vi "בדיקת מפל מתח בין הדקי הממסר תחת עומס 7.vi"(8 "error":errorcluster, 11 "Path for Log":path) -> (0 "error IO":errorcluster, 1 "בטווח כן/לא":bool, 2 "מפל מתח בין דקי הממסר תחת עומס":dbl, 3 "תוצאה זמנית":dbl)   [LabVIEW 2014]
uses:
  M9700 Driver/85/vi.lib/M9700 Modbus.llb/CTL Register Address.ctl
  M9700 Driver/86/vi.lib/M9700 Modbus.llb/CTL CMD Register.ctl
  <vilib>/Instr/_visa.llb/VISA Configure Serial Port (Instr).vi
  <vilib>/DAQmx/create/channels.llb/DAQmx Create Channel (DO-Digital Output).vi
  <vilib>/DAQmx/write.llb/DAQmx Write (Digital Bool 1Line 1Point).vi
panel:
  out "progress":dbl(slide) min=0.0 max=10.0 scale=0.0..10.0
  in  "stop":bool
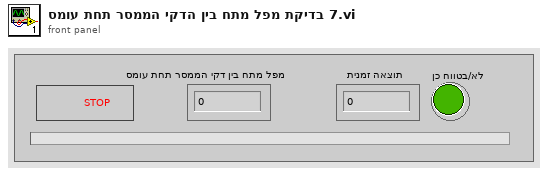
[diagram p1: front panel]
types:
  T1 = enum32{"Invalid", "Standard", "Closed", "Hidden", "Minimized", "Maximized"}
  T2 = typedef "CTL CMD Register.ctl" = u8
  T3 = typedef "CTL Register Address.ctl" = u16
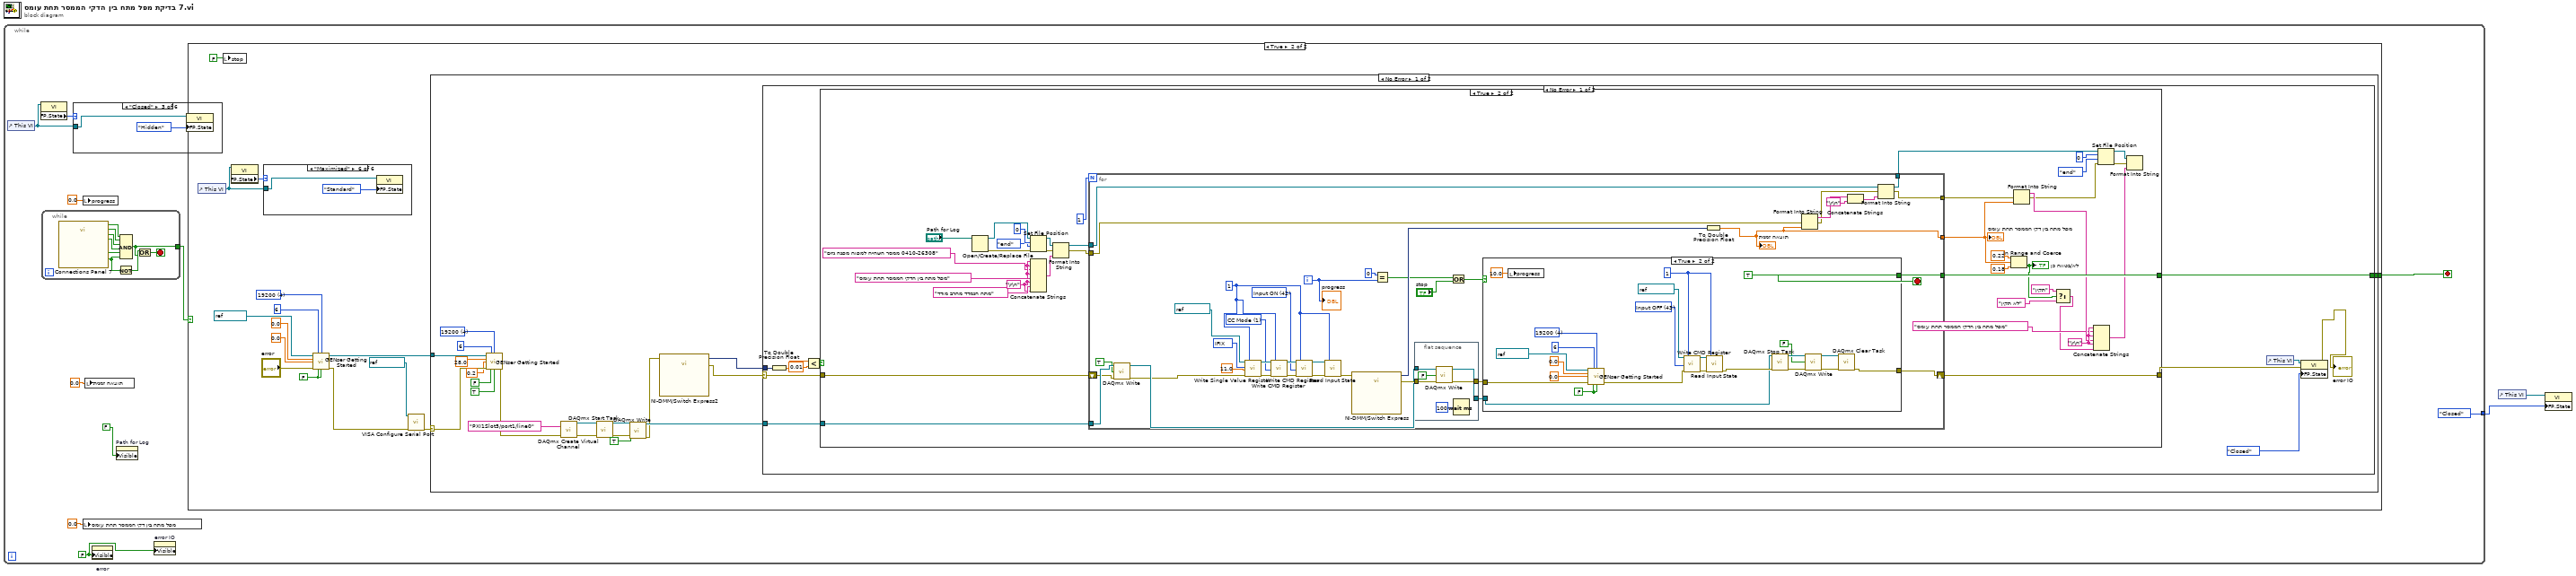
[diagram p0: block diagram]
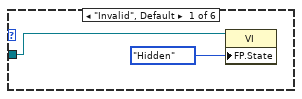
[diagram p2: hidden frame]
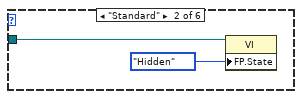
[diagram p3: hidden frame]
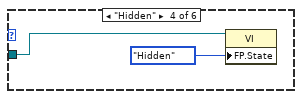
[diagram p4: hidden frame]
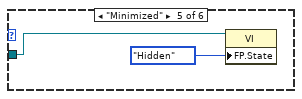
[diagram p5: hidden frame]
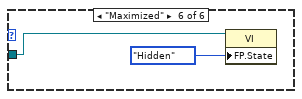
[diagram p6: hidden frame]
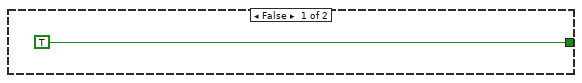
[diagram p7: hidden frame]
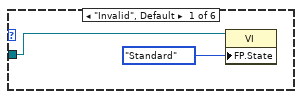
[diagram p8: hidden frame]
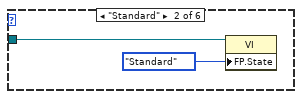
[diagram p9: hidden frame]
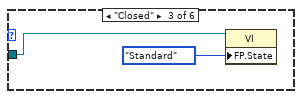
[diagram p10: hidden frame]
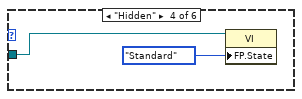
[diagram p11: hidden frame]
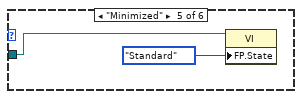
[diagram p12: hidden frame]
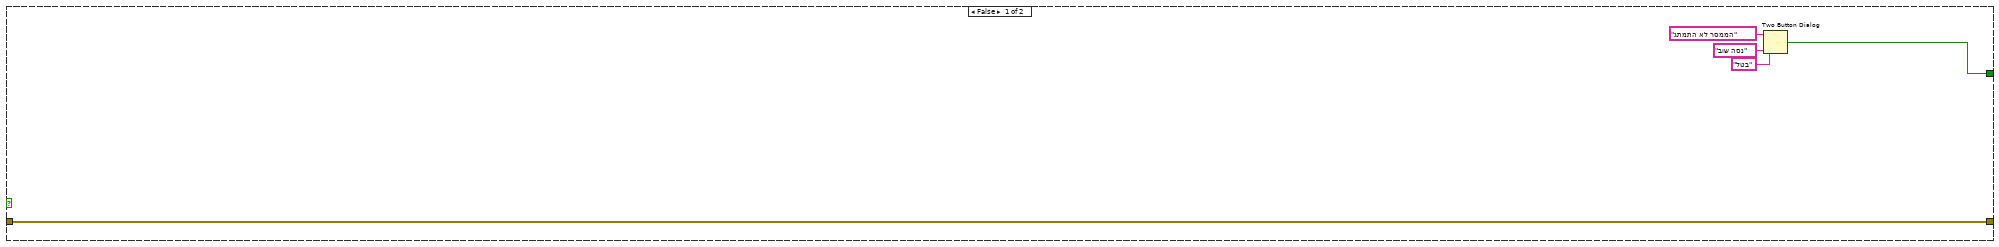
[diagram p13: hidden frame]
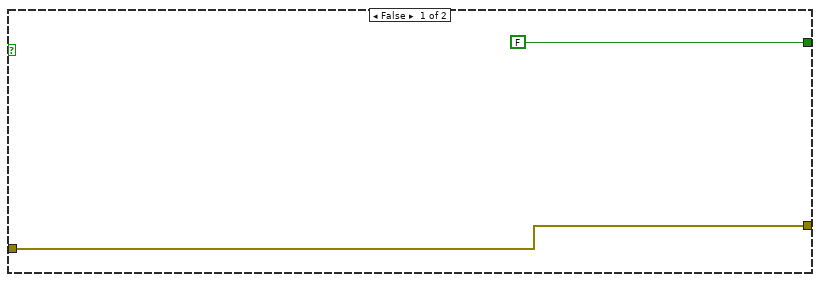
[diagram p14: hidden frame]
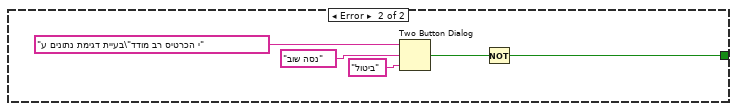
[diagram p15: hidden frame]
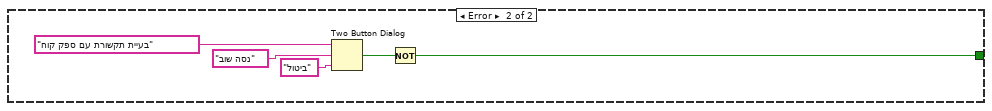
[diagram p16: hidden frame]
diagram:
  n1 = while {
    tunnel: [T1."Closed" ("Front Panel Window:State")] -> w1
    stop <- w12 stop-if-true
    w8 = FALSE ("Visible")
    n2 = control-ref of="This VI"() -> (w5:refnum<vi>)
    n3 = property class="VI"(reference=w5) -> ("FP.State"=w4:T1)  [unwired: 1 in, 2 out]
    n4 = while {
      tunnel: [w13] -> w6
      stop <- w16 stop-if-true
      n5 = call "Connections Panel 7.vi"() -> ("Input Name 10"=w17:bool, "Input Name 6"=w21:bool, "Input Name 7"=w20:bool, "Input Name 8"=w19:bool, "Input Name 9"=w18:bool, "OK"=w14:bool)  [unwired: 13 in, 1 out]
      n6 = Not(x=w14) -> (.not. x?=w15:bool)
      n7 = Compound Arithmetic op=AND(w21, w20, w19, w18, w17, w14) -> (w13:bool)
      n8 = Or(x=w15, y=w13) -> (x .or. y?=w16:bool)
    }
    n9 = case shown="\"Closed\"" w4 {
      tunnel: w5 -> [w22 w24 w26 w28 w30 w32]
      frame "Invalid", Default {
        n10 = property class="VI"(reference=w22, "FP.State"=T1."Hidden" ("Front Panel Window:State")) -> ()  [unwired: 1 in, 2 out]
      }
      frame "Standard" {
        n11 = property class="VI"(reference=w24, "FP.State"=T1."Hidden" ("Front Panel Window:State")) -> ()  [unwired: 1 in, 2 out]
      }
      frame "Closed" {
        n12 = property class="VI"(reference=w26, "FP.State"=T1."Hidden" ("Front Panel Window:State")) -> ()  [unwired: 1 in, 2 out]
      }
      frame "Hidden" {
        n13 = property class="VI"(reference=w28, "FP.State"=T1."Hidden" ("Front Panel Window:State")) -> ()  [unwired: 1 in, 2 out]
      }
      frame "Minimized" {
        n14 = property class="VI"(reference=w30, "FP.State"=T1."Hidden" ("Front Panel Window:State")) -> ()  [unwired: 1 in, 2 out]
      }
      frame "Maximized" {
        n15 = property class="VI"(reference=w32, "FP.State"=T1."Hidden" ("Front Panel Window:State")) -> ()  [unwired: 1 in, 2 out]
      }
    }
    n16 = local write "progress"(0.0 ("progress")) -> ()
    n17 = local write "מפל מתח בין דקי הממסר תחת עומס"(0.0 ("מפל מתח בין דקי הממסר תחת עומס")) -> ()
    n18 = local write "תוצאה זמנית"(0.0 ("תוצאה זמנית")) -> ()
    n19 = property on="error" class="Clust (strict)"("Visible"=w8) -> ()  [unwired: 2 in, 2 out]
    n20 = property on="Path for Log" class="Path"("Visible"=FALSE) -> ()  [unwired: 2 in, 2 out]
    n21 = property on="error IO" class="Clust (strict)"("Visible"=w8) -> ()  [unwired: 2 in, 2 out]
    n22 = case shown="True" w6 {
      tunnel: [TRUE w42] -> w12
      frame False {
      }
      frame True {
        w39 = FALSE ("Output On (T)")
        w46 = u16 4 items=["1200", "2400", "4800", "9600", "19200"] ("BAUD")
        n23 = control-ref of="This VI"() -> (w36:refnum<vi>)
        n24 = local write "stop"(FALSE ("stop")) -> ()
        n25 = property class="VI"(reference=w36) -> ("FP.State"=w37:T1)  [unwired: 1 in, 2 out]
        n26 = case shown="\"Maximized\"" w37 {
          tunnel: w36 -> [w50 w52 w54 w56 w58 w60]
          frame "Invalid", Default {
            n27 = property class="VI"(reference=w50, "FP.State"=T1."Standard" ("Front Panel Window:State")) -> ()  [unwired: 1 in, 2 out]
          }
          frame "Standard" {
            n28 = property class="VI"(reference=w52, "FP.State"=T1."Standard" ("Front Panel Window:State")) -> ()  [unwired: 1 in, 2 out]
          }
          frame "Closed" {
            n29 = property class="VI"(reference=w54, "FP.State"=T1."Standard" ("Front Panel Window:State")) -> ()  [unwired: 1 in, 2 out]
          }
          frame "Hidden" {
            n30 = property class="VI"(reference=w56, "FP.State"=T1."Standard" ("Front Panel Window:State")) -> ()  [unwired: 1 in, 2 out]
          }
          frame "Minimized" {
            n31 = property class="VI"(reference=w58, "FP.State"=T1."Standard" ("Front Panel Window:State")) -> ()  [unwired: 1 in, 2 out]
          }
          frame "Maximized" {
            n32 = property class="VI"(reference=w60, "FP.State"=T1."Standard" ("Front Panel Window:State")) -> ()  [unwired: 1 in, 2 out]
          }
        }
        n33 = call "GENser Getting Started.vi"("VISA"=refnum<visa-resource-name> "COM6", "GEN Addr"=i16 6, "BAUD"=w46, "Voltage Limit"=0.0, "Current Limit"=0.0, "error"="error", "Reset (T)"=w39, "Output On (T)"=w39) -> ("VISA out"=w48:refnum<visa-resource-name>, "error out"=w35:errorcluster)  [unwired: 4 in, 2 out]
        n34 = call-poly "VISA Configure Serial Port"("VISA resource name"=refnum<visa-resource-name> "COM13", "error in (no error)"=w35) -> ("error out"=w40:errorcluster)  [unwired: 4 in, 9 out]
        n35 = case shown="No Error" w40 {
          selector: w40 -> [w78 _]
          tunnel: w48 -> [w81 _]
          tunnel: [w80 w209] -> w42
          frame No Error {
            w72 = u16 4 items=["1200", "2400", "4800", "9600", "19200"] ("BAUD")
            n36 = call "GENser Getting Started.vi"("VISA"=w81, "GEN Addr"=i16 6, "BAUD"=w72, "Voltage Limit"=28.0, "Current Limit"=0.2, "error"=w78, "Reset (T)"=FALSE, "Output On (T)"=TRUE) -> ("error out"=w67:errorcluster)  [unwired: 4 in, 3 out]
            n37 = call-poly <vilib>:"DAQmx Create Virtual Channel.vi"("lines"=tag "PXI1Slot5/port1/line0", "error in"=w67) -> ("task out"=w70:refnum<k21>, "error out"=w71:errorcluster)  [unwired: 12 in]
            n38 = call <vilib>:"DAQmx Start Task.vi"("task/channels in"=w70, "error in"=w71) -> ("task out"=w66:refnum<k21>, "error out"=w64:errorcluster)  [unwired: 12 in]
            n39 = call-poly <vilib>:"DAQmx Write.vi"("task/channels in"=w66, "data"=TRUE, "error in"=w64) -> ("task out"=w65:refnum<k21>, "error out"=w63:errorcluster)  [unwired: 10 in, 1 out]
            n40 = call "NI-DMM/Switch Express2"("error in"=w63) -> ("signals out"=w79:dynamicdata, "error out"=w68:errorcluster)  [unwired: 16 in, 1 out]
            n41 = case shown="No Error" w68 {
              selector: w68 -> [w90 _]
              tunnel: [w89 w204] -> w80
              tunnel: w79 -> [w92 _]
              tunnel: w65 -> [w83 _]
              frame No Error {
                n42 = To Double Precision Float(number=w92) -> (double precision float=w88:dbl)
                n43 = Less?(x=w88, y=0.01) -> (x < y?=w91:bool)
                n44 = case shown="True" w91 {
                  tunnel: w90 -> [w97 w132]
                  tunnel: [w93 w133] -> w89
                  tunnel: [w97 w128] -> w84
                  tunnel: w83 -> [_ w129]
                  frame False {
                    n45 = Two Button Dialog(message="הממסר לא התמתג", 1:"נסה שוב" ("F button name (\"Cancel\")"), 2:"בטל" ("T button name (\"OK\")")) -> (T button?=w93:bool)
                  }
                  frame True {
                    w114 = "\r\n"
                    w117 = "\r\n"
                    n46 = Open/Create/Replace File(file path (use dialog)="Path for Log") -> (refnum out=w125:refnum<file>, error out=w124:errorcluster)  [unwired: 5 in, 1 out]
                    n47 = Set File Position(offset (in bytes) (0)=i64 0, refnum=w125, from (0:start)=enum16{"start", "end", "current"}."end", error in=w124) -> (refnum out=w121:refnum<file>, error out=w118:errorcluster)
                    n48 = Concatenate Strings(w117, w117, "ממסר השהייה למפוח מפנה גזים 0410-26308", w117, "מפל מתח בין הדקי הממסר תחת עומס", w117, "מתח הנמדד מהרב מודד", w117) -> (w123:string)
                    n49 = Format Into String(initial string=w121, error in=w118, w123) -> (resulting string=w115:refnum<file>, error out=w116:errorcluster)  [unwired: 1 in]
                    n50 = for {
                      N: 1 -> [_]
                      tunnel: [w155] -> w133
                      shift-right: [w153] -> w128
                      shift-left: w132 -> [w148]
                      tunnel: w129 -> [w149]
                      tunnel: w116 -> [w139]
                      tunnel: w115 -> [w141]
                      tunnel: [w138] -> w108
                      tunnel: [w137] -> w100
                      tunnel: [w136] -> w98
                      i -> [w152]
                      stop <- w155 stop-if-true
                      w163 = T2 42 items=["CC Mode"=1, "CV Mode"=2, "CW Mode"=3, "CR Mode"=4, "Short Mode"=26, "Set SysPara"=41, "Input ON"=42, "Input OFF"=43] ("CMD Register Value")
                      w166 = u8 1 ("Load Address")
                      w169 = T2 1 items=["CC Mode"=1, "CV Mode"=2, "CW Mode"=3, "CR Mode"=4, "Short Mode"=26, "Set SysPara"=41, "Input ON"=42, "Input OFF"=43] ("CMD Register Value")
                      w172 = T3 2561 items=["REMOTE"=1283, "ISTATE"=1296, "CMD"=2560, "IFIX"=2561, "UFIX"=2563, "PFIX"=2565, "RFIX"=2567, "IMAX"=2612, "UMAX"=2614, "PMAX"=2616, "U"=2816, "I"=2818, "MODEL"=2822, "EDITION"=2823] ("Register Address")
                      n51 = call-poly <vilib>:"DAQmx Write.vi"("task/channels in"=w149, "data"=TRUE, "error in"=w148) -> ("task out"=w147:refnum<k21>, "error out"=w135:errorcluster)  [unwired: 10 in, 1 out]
                      n52 = call "Write Single Value Register.vi"("VISA resource name"=refnum<visa-resource-name> "COM13", "Starting Address(HEX)"=w172, "Register Single Value"=sgl 11.0, "error in"=w135, "Load Address"=w166) -> ("VISA resource name out"=w171:refnum<visa-resource-name>, "error out"=w170:errorcluster)  [unwired: 13 out]
                      n53 = call "Write CMD Register.vi"("VISA resource name"=w171, "CMD Value"=w169, "error in"=w170, "Load Address"=w166) -> ("VISA resource name out"=w167:refnum<visa-resource-name>, "error out"=w164:errorcluster)  [unwired: 14 out]
                      n54 = call "Write CMD Register.vi"("VISA resource name"=w167, "CMD Value"=w163, "error in"=w164, "Load Address"=w166) -> ("VISA resource name out"=w165:refnum<visa-resource-name>, "error out"=w162:errorcluster)  [unwired: 14 out]
                      n55 = call "Read Input State.vi"("VISA resource name"=w165, "error in"=w162, "Load Address"=w166) -> ("error out"=w161:errorcluster)  [unwired: 16 out]
                      n56 = call "NI-DMM/Switch Express"("error in"=w161) -> ("signals out"=w160:dynamicdata, "error out"=w150:errorcluster)  [unwired: 16 in, 1 out]
                      n57 = Equal?(x=0, y=w152) -> (x = y?=w157:bool)
                      n58 = flat-sequence {
                        tunnel: [w178] -> w151
                        tunnel: w150 -> [w177]
                        tunnel: w147 -> [w175]
                        tunnel: [w174] -> w145
                        frame #0 {
                          n59 = call-poly <vilib>:"DAQmx Write.vi"("task/channels in"=w175, "data"=FALSE, "error in"=w177) -> ("task out"=w174:refnum<k21>, "error out"=w178:errorcluster)  [unwired: 10 in, 1 out]
                          n60 = Wait (ms)(milliseconds to wait=u32 100) -> ()  [unwired: 1 out]
                        }
                      }
                      n61 = Or(x=w157, y="stop") -> (x .or. y?=w158:bool)
                      n62 = case shown="True" w158 {
                        tunnel: [FALSE TRUE] -> w155
                        tunnel: w151 -> [w179 w197]
                        tunnel: [w179 w183] -> w153
                        tunnel: w145 -> [_ w182]
                        frame False {
                        }
                        frame True {
                          w191 = u8 1 ("Load Address")
                          w194 = T2 43 items=["CC Mode"=1, "CV Mode"=2, "CW Mode"=3, "CR Mode"=4, "Short Mode"=26, "Set SysPara"=41, "Input ON"=42, "Input OFF"=43] ("CMD Register Value")
                          w196 = FALSE ("Reset (T)")
                          w199 = u16 4 items=["1200", "2400", "4800", "9600", "19200"] ("BAUD")
                          n63 = local write "progress"(10.0 ("progress")) -> ()
                          n64 = call "GENser Getting Started.vi"("VISA"=refnum<visa-resource-name> "COM6", "GEN Addr"=i16 6, "BAUD"=w199, "Voltage Limit"=0.0, "Current Limit"=0.0, "error"=w197, "Reset (T)"=w196, "Output On (T)"=w196) -> ("error out"=w181:errorcluster)  [unwired: 4 in, 3 out]
                          n65 = call "Write CMD Register.vi"("VISA resource name"=refnum<visa-resource-name> "COM13", "CMD Value"=w194, "error in"=w181, "Load Address"=w191) -> ("VISA resource name out"=w192:refnum<visa-resource-name>, "error out"=w195:errorcluster)  [unwired: 14 out]
                          n66 = call "Read Input State.vi"("VISA resource name"=w192, "error in"=w195, "Load Address"=w191) -> ("error out"=w184:errorcluster)  [unwired: 16 out]
                          n67 = call <vilib>:"DAQmx Stop Task.vi"("task/channels in"=w182, "error in"=w184) -> ("task out"=w189:refnum<k21>, "error out"=w187:errorcluster)  [unwired: 12 in]
                          n68 = call-poly <vilib>:"DAQmx Write.vi"("task/channels in"=w189, "data"=FALSE, "error in"=w187) -> ("task out"=w186:refnum<k21>, "error out"=w185:errorcluster)  [unwired: 10 in, 1 out]
                          n69 = call <vilib>:"DAQmx Clear Task.vi"("task in"=w186, "error in"=w185) -> ("error out"=w183:errorcluster)  [unwired: 13 in]
                        }
                      }
                      n70 = To Double Precision Float(number=w160) -> (double precision float=w136:dbl)
                      "תוצאה זמנית" <- w136
                      n71 = Format Into String(error in=w139, w136) -> (resulting string=w143:string, error out=w140:errorcluster)  [unwired: 2 in]
                      n72 = Concatenate Strings(w143, "\r\n") -> (w142:string)
                      n73 = Format Into String(initial string=w141, error in=w140, w142) -> (resulting string=w138:refnum<file>, error out=w137:errorcluster)  [unwired: 1 in]
                      "progress" <- w152
                    }
                    "מפל מתח בין דקי הממסר תחת עומס" <- w98
                    n74 = In Range and Coerce(upper limit=0.22, x=w98, lower limit=0.18) -> (In Range?=w103:bool)  [unwired: 1 out]
                    "בטווח כן/לא" <- w103
                    n75 = Format Into String(error in=w100, w98) -> (resulting string=w107:string, error out=w101:errorcluster)  [unwired: 2 in]
                    n76 = Select(t="תקין", s=w103, f="לא תקין") -> (s? t:f=w102:string)
                    n77 = Concatenate Strings(w114, "מפל מתח בין הדקי הממסר תחת עומס" ("string"), w114, w107, w114, w102) -> (w109:string)
                    n78 = Set File Position(offset (in bytes) (0)=i64 0, refnum=w108, from (0:start)=enum16{"start", "end", "current"}."end", error in=w101) -> (refnum out=w111:refnum<file>, error out=w110:errorcluster)
                    n79 = Format Into String(initial string=w111, error in=w110, w109) -> ()  [unwired: 1 in, 2 out]
                  }
                }
                n80 = control-ref of="This VI"() -> (w86:refnum<vi>)
                n81 = property class="VI"(reference=w86, error in=w84, "FP.State"=T1."Closed" ("Front Panel Window:State")) -> (error out=→"error IO":errorcluster)  [unwired: 1 out]
              }
              frame Error {
                n82 = Two Button Dialog(message="בעיית דגימת נתונים ע\"י הכרטיס רב מודד", 1:"ביטול" ("F button name (\"Cancel\")"), 2:"נסה שוב" ("T button name (\"OK\")")) -> (T button?=w205:bool)
                n83 = Not(x=w205) -> (.not. x?=w204:bool)
              }
            }
          }
          frame Error {
            n84 = Two Button Dialog(message="בעיית תקשורת עם ספק קוח", 1:"ביטול" ("F button name (\"Cancel\")"), 2:"נסה שוב" ("T button name (\"OK\")")) -> (T button?=w210:bool)
            n85 = Not(x=w210) -> (.not. x?=w209:bool)
          }
        }
      }
    }
  }
  n86 = control-ref of="This VI"() -> (w2:refnum<vi>)
  n87 = property class="VI"(reference=w2, "FP.State"=w1) -> ()  [unwired: 1 in, 2 out]
